vi "Client.vi"() -> ()   [LabVIEW 2015]
panel:
  out "data in":string="Hello World!"
  in  "stop":bool
  out "error out":errorcluster
  in  "error in (no error)":errorcluster
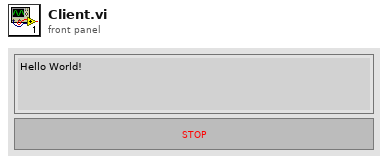
[diagram p1: front panel]
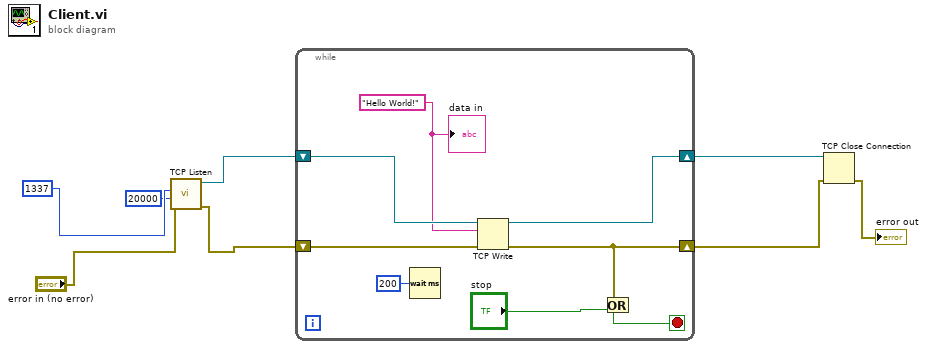
[diagram p0: block diagram]
diagram:
  n1 = call <vilib>:"TCP Listen.vi"("error in (no error)"="error in (no error)", "timeout ms (wait forever: -1)"=20000, "port"=1337 ("timeout ms (60000)")) -> ("error out"=w2:errorcluster, "connection ID"=w4:refnum<k5>)  [unwired: 4 in, 3 out]
  n2 = while {
    shift-right: [w14] -> w8
    shift-left: w4 -> [w16]
    shift-right: [w11] -> w7
    shift-left: w2 -> [w15]
    stop <- w13 stop-if-true
    w9 = "Hello World!" ("data in")
    n3 = Wait (ms)(milliseconds to wait=u32 200) -> ()  [unwired: 1 out]
    n4 = TCP Write(connection ID=w16, data in=w9, error in (no error)=w15) -> (connection ID out=w14:refnum<k5>, error out=w11:errorcluster)  [unwired: 1 in, 1 out]
    n5 = Or(x=w11, y="stop") -> (x .or. y?=w13:bool)
    "data in" <- w9
  }
  n6 = TCP Close Connection(connection ID=w8, error in (no error)=w7) -> (error out=→"error out":errorcluster)  [unwired: 1 in, 1 out]
